vi "SDG60UploadArbWaveform2.vi"(3 "WFM (Column) Number":i32, 5 "WFM Numer ARBn":u32=1, 9 "Timeout (40000 ms)":u32=40000, 13 "Number of retries":i32=1, 14 "WFM Source":u16(ring) items=["Single file", "Split files", "Array"]) -> (10 "Total time":dbl format="%#_15g")   [LabVIEW 2022 SP3]
doc: "Creates and saves an arbitrary (user-defined) waveform in non-volatile memory, then selects it for output."
uses:
  <vilib>/addons/zeromq/socket_type.ctl
  <vilib>/addons/zeromq/zmq_context.lvclass
  <vilib>/addons/zeromq/zmq_socket.lvclass
  <vilib>/addons/zeromq/zeromq.lvlib
panel:
  in  "Load to output":bool
  out "Python response":string
  out "WFM (Column) Number imdicator":i32
  out "WFM Source indciator":u16(ring) items=["Single file", "Split files", "Array"]
  out "Time at end":timestamp
  out "Time at start":timestamp
  out "Upload time":dbl format="%#_15g"
  out "Attempts (0: First)":i32
  in  "WFM Path":path=path "C:/Data/_SoftDevelopment/SDG6000/WFMTst20E6PtsInt.txt"
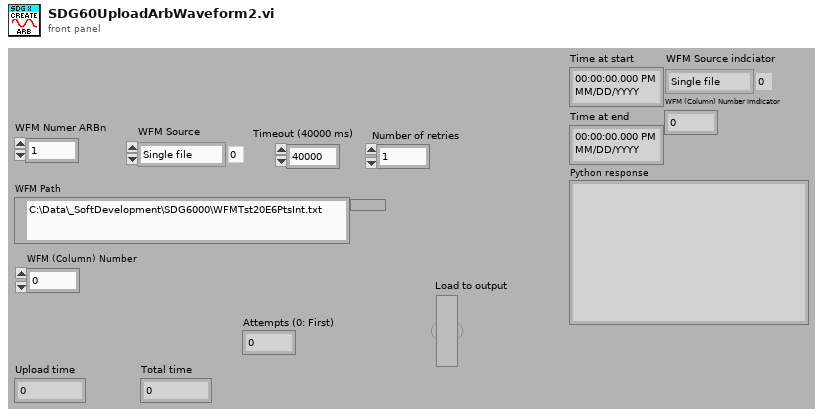
[diagram p1: front panel]
types:
  T1 = typedef "zeromq.lvlib/socket_type.ctl" = enum8{"ZMQ_PAIR", "ZMQ_PUB", "ZMQ_SUB", "ZMQ_REQ", "ZMQ_REP", "ZMQ_DEALER", "ZMQ_ROUTER", "ZMQ_PULL", "ZMQ_PUSH", "ZMQ_XPUB", "ZMQ_XSUB", "ZMQ_STREAM", "ZMQ_SERVER", "ZMQ_CLIENT", "ZMQ_RADIO", "ZMQ_DISH", "ZMQ_GATHER", "ZMQ_SCATTER", "ZMQ_DGRAM"}
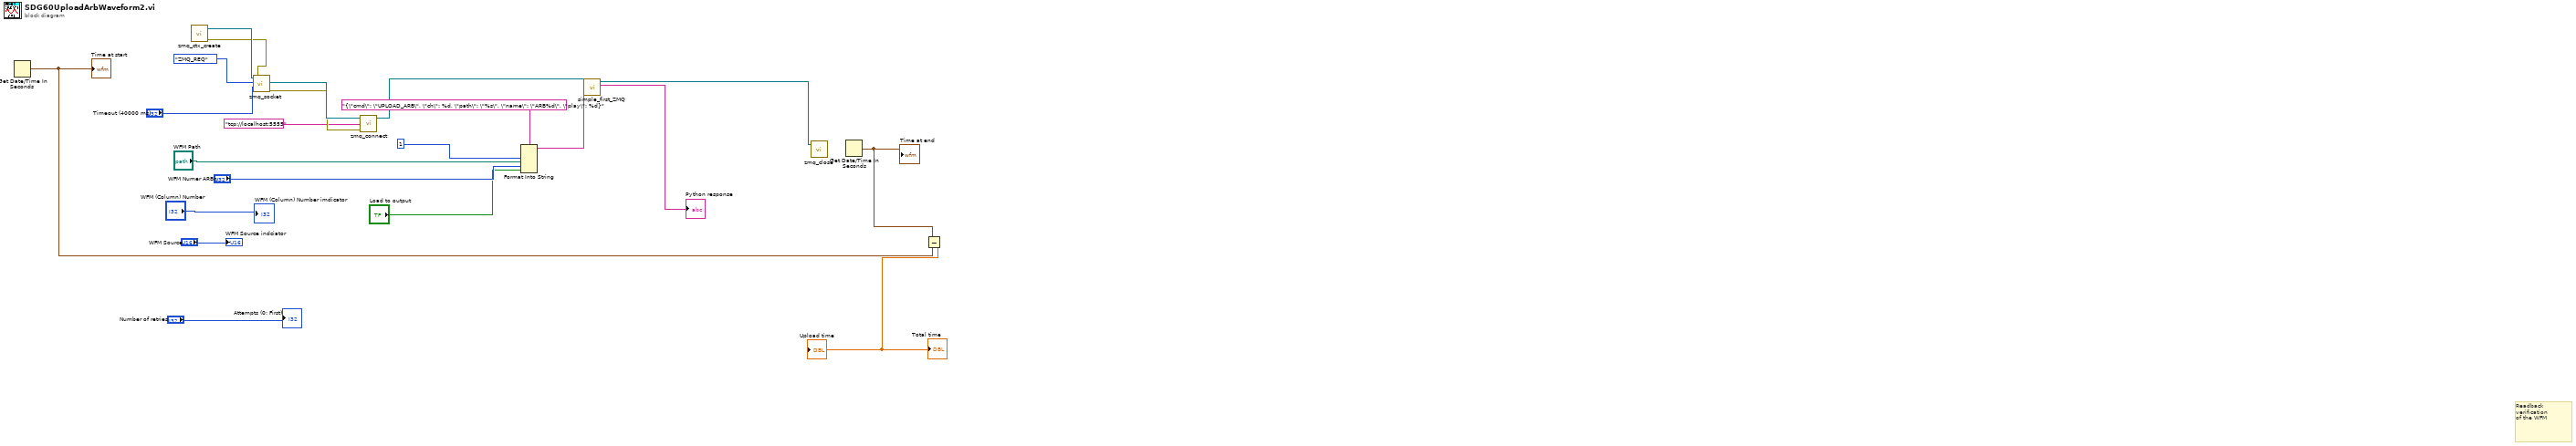
[diagram p0: block diagram]
diagram:
  # "Readback verification\nof the WFM"
  n1 = Get Date/Time In Seconds() -> (seconds since 1Jan1904=w4:timestamp)
  "Time at start" <- w4
  n2 = call <vilib>:"zmq_ctx_create.vi"() -> ("error out"=w14:errorcluster, "context out"=w16:refnum<class "zmq_context.lvclass">)  [unwired: 4 in]
  n3 = call <vilib>:"zmq_socket.vi"("error in"=w14, "linger (ms)"="Timeout (40000 ms)", "socket type"=socket_type."ZMQ_REQ", "context in"=w16) -> ("error out"=w13:errorcluster, "socket out"=w15:refnum<class "zmq_socket.lvclass">)  [unwired: 1 in, 1 out]
  n4 = call <vilib>:"zmq_connect.vi"("error in"=w13, "endpoint"="tcp://localhost:5555", "socket in"=w15) -> ("socket out"=w10:refnum<class "zmq_socket.lvclass">)  [unwired: 1 in, 1 out]
  n5 = Format Into String(format string="{\"cmd\": \"UPLOAD_ARB\", \"ch\": %d, \"path\": \"%s\", \"name\": \"ARB%d\", \"play\": %d}", u32 1 ("input 1"), "WFM Path", "WFM Numer ARBn", "Load to output") -> (resulting string=w7:string)  [unwired: 2 in, 1 out]
  n6 = call "simple_first_ZMQ.vi"("Raw command"=w7, "ZMQ socket in"=w10) -> ("Python response"=→"Python response":string, "ZMQ socket out"=w9:refnum<class "zmq_socket.lvclass">)  [unwired: 4 in]
  n7 = call <vilib>:"zmq_close.vi"("socket"=w9) -> ()  [unwired: 4 in, 1 out]
  n8 = Get Date/Time In Seconds() -> (seconds since 1Jan1904=w3:timestamp)
  "Time at end" <- w3
  n9 = Subtract(x=w4, y=w3) -> (x-y=→"Total time" →"Upload time":dbl)
  "Attempts (0: First)" <- "Number of retries"
  "WFM Source indciator" <- "WFM Source"
  "WFM (Column) Number imdicator" <- "WFM (Column) Number"
